vi "Launch Configured Tasks.vi"(8 "error in (no error)":errorcluster, 11 "Volatus Core in":refnum<class "Volatus Core.lvclass">) -> (0 "error out":errorcluster, 3 "Volatus Core out":refnum<class "Volatus Core.lvclass">)   [LabVIEW 2020, in "Volatus.lvlib" / "Volatus Core.lvclass"]
uses:
  Volatus Core.lvclass
  Volatus Core.lvclass/Volatus Core.ctl
  VolatusAPI/VolatusAPI.lvclass
  Module/Module.lvclass
  VolatusConfig/Node/Node.lvclass
  VolatusConfig/Task/Task.lvclass
  C:/dev/lv20CE/relink/lv-volatus/VolatusConfig/VolatusConfigElement/VolatusConfigElement.lvclass
  C:/dev/lv20CE/relink/lv-volatus/VolatusConfig/Task/Task.lvclass
  C:/dev/lv20CE/relink/lv-volatus/Volatus/Module/Module.lvclass
  C:/dev/lv20CE/relink/lv-volatus/Volatus/Volatus Core/Volatus Core.lvclass
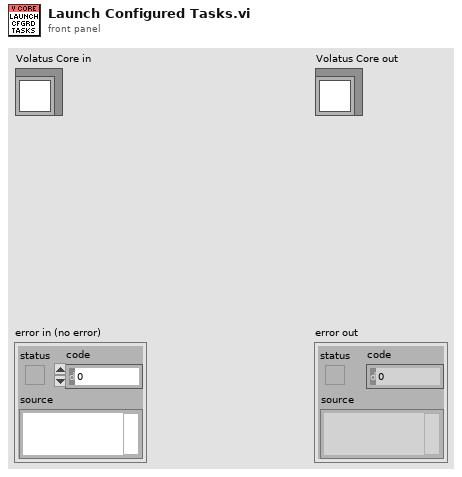
[diagram p1: front panel]
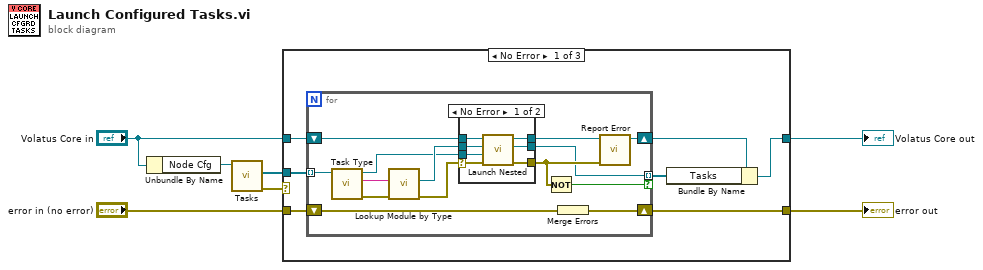
[diagram p0: block diagram]
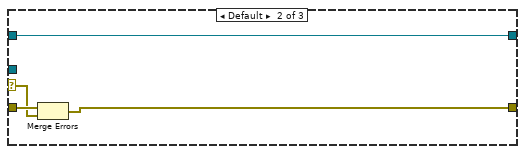
[diagram p3: hidden frame]
diagram:
  n1 = Unbundle By Name("Volatus Core in") -> ("Node Cfg"=w6:refnum<class "Node.lvclass">)
  n2 = call "Tasks.vi"("Node in"=w6) -> ("error out"=w1:errorcluster, "Tasks"=w5:refnum<class "Task.lvclass">[])  [unwired: 8 in, 1 out]
  n3 = case shown="No Error" w1 {
    selector: w1 -> [_ w39 _]
    tunnel: [w14 w38 w43] -> w7
    tunnel: w5 -> [w12 _ _]
    tunnel: "error in (no error)" -> [w11 w40 w43]
    tunnel: "Volatus Core in" -> [w10 w41 w42]
    tunnel: [w9 w41 w42] -> w2
    frame No Error {
      n4 = for {
        tunnel: w12 -> [w21] mode=indexing
        shift-right: [w15] -> w13
        shift-left: w10 -> [w27]
        shift-right: [w22] -> w14
        shift-left: w11 -> [w23]
        tunnel: [w17] -> w8 mode=indexing if=w16
        n5 = call "Task Type.vi"("Task in"=w21) -> ("error out"=w18:errorcluster, "Task Type"=w19:string, "Task out"=w20:refnum<class "Task.lvclass">)  [unwired: 8 in]
        n6 = call "Lookup Module by Type.vi"("error in (no error)"=w18, "Module Type"=w19) -> ("error out"=w25:errorcluster, "Module Type"=w26:refnum<class "Module.lvclass">)  [unwired: 8 in]
        n7 = case shown="No Error" w25 {
          selector: w25 -> [w32 w36]
          tunnel: w27 -> [w35 w37]
          tunnel: w26 -> [w34 _]
          tunnel: w20 -> [w33 _]
          tunnel: [w31 w36] -> w28
          tunnel: [w30 w37] -> w24
          tunnel: [w29 _] -> w17
          frame No Error {
            n8 = call "Launch Nested.vi"("error in (no error)"=w32, "Config Element"=w33, "Nested Module"=w34, "Parent in"=w35) -> ("error out"=w31:errorcluster, "MessageQ"=w29:refnum<class "MessageQ.lvclass">, "Parent out"=w30:refnum<class "Volatus Core.lvclass">)  [unwired: 5 in]
          }
          frame Error {
          }
        }
        n9 = Not(x=w28) -> (.not. x?=w16:bool)
        n10 = Merge Errors(w23) -> (w22:errorcluster)
        n11 = call "Report Error.vi"("error in (no error)"=w28, "Module in"=w24) -> ("Module out"=w15:refnum<class "Volatus Core.lvclass">)  [unwired: 8 in, 1 out]
      }
      n12 = Bundle By Name(cluster=w13, "Tasks"=w8) -> (w9:refnum<class "Volatus Core.lvclass">)
    }
    frame Default {
      n13 = Merge Errors(w40, w39) -> (w38:errorcluster)
    }
    frame Error {
      # "Tasks entry not present, this can be the case for command server apps, though eventually those will have a status GUI. Also for unconfigured systems."
    }
  }
  "error out" <- w7
  "Volatus Core out" <- w2
